vi "Create_Event_ToHmiScheduler.vi"(8 "error in (no error)":errorcluster, 11 "EVE reference in":refnum<data-value>) -> (0 "error out":errorcluster, 3 "EVE reference out":refnum<data-value>)   [LabVIEW 2013, in "EVE.lvclass"]
uses:
  EVE.lvclass
  030 - EVENTS/EnumFgvEventCommand.ctl
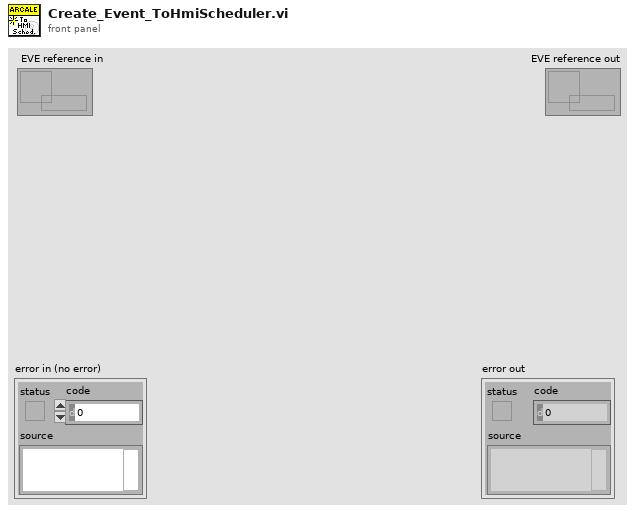
[diagram p1: front panel]
types:
  T1 = typedef "EnumFgvEventCommand.ctl" = enum16{"Setup", "Cleanup", "Get"}
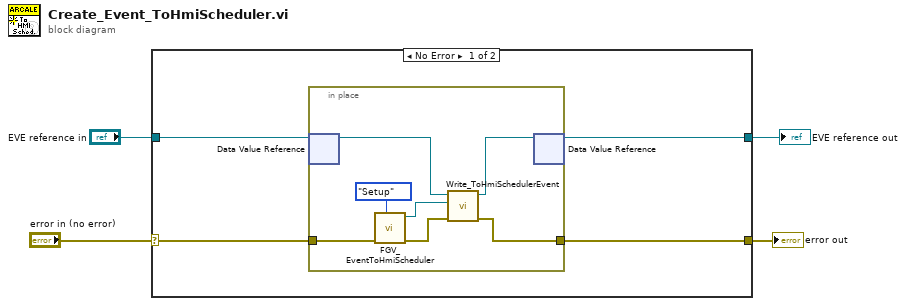
[diagram p0: block diagram]
diagram:
  n1 = case shown="No Error" "error in (no error)" {
    selector: "error in (no error)" -> [w8 w17]
    tunnel: [w7 w17] -> w3
    tunnel: "EVE reference in" -> [w6 w16]
    tunnel: [w5 w16] -> w1
    frame No Error {
      n2 = in-place {
        in-place-border: w8 -> [w12]
        in-place-border: [w11] -> w7
        n3 = in-place-dvr #1(w6) -> (w10:refnum<class "EVE.lvclass">)  [unwired: 1 out]
        n4 = call "FGV_EventToHmiScheduler.vi"("Command"=EnumFgvEventCommand."Setup", "error in (no error)"=w12) -> ("error out"=w13:errorcluster, "ToHmiSchedulerEvent"=w14:refnum<user-event>)  [unwired: 8 in]
        n5 = call-dynamic "Write_ToHmiSchedulerEvent.vi"("error in (no error)"=w13, "ToHmiSchedulerEvent"=w14, "EVE in"=w10) -> ("error out"=w11:errorcluster, "EVE out"=w9:refnum<class "EVE.lvclass">)  [unwired: 7 in]
        n6 = in-place-dvr #1(w9) -> (w5:refnum<data-value>)  [unwired: 1 out]
      }
    }
    frame Error {
    }
  }
  "error out" <- w3
  "EVE reference out" <- w1
